vi "Initialize.vi"(8 "error in (no error)":errorcluster, 10 "timeout (ms)":u32=10000, 11 "VISA resource name":refnum<visa-resource-name>) -> (0 "error out":errorcluster, 3 "reference out":refnum<visa-resource-name>)   [LabVIEW 2012, in "USGlobalSat.lvlib"]
uses:
  USGlobalSat.lvlib
  <vilib>/Instr/_visa.llb/VISA Configure Serial Port (Instr).vi
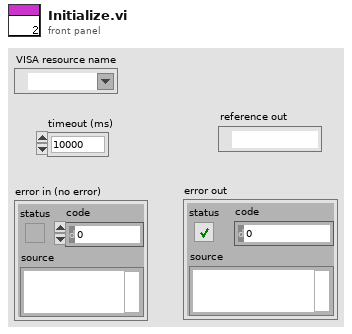
[diagram p1: front panel]
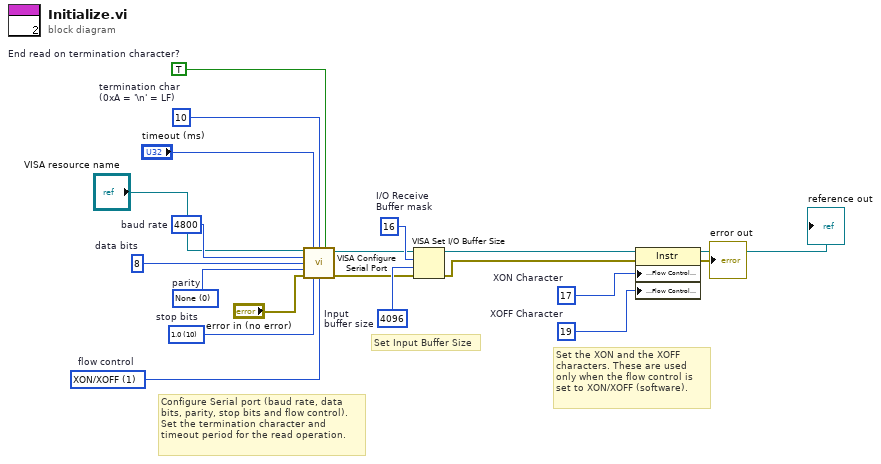
[diagram p0: block diagram]
diagram:
  w16 = TRUE  # End read on termination character?
  w8 = u8 19  # XOFF Character
  w9 = u8 17  # XON Character
  w14 = u32 4096  # Input buffer size
  w12 = u16 1 items=["None"=0, "XON/XOFF"=1, "RTS/CTS"=2, "DTR/DSR"=4]  # flow control
  w18 = u16 10 items=["1.0"=10, "1.5"=15, "2.0"=20]  # stop bits
  w19 = u16 0 items=["None", "Odd", "Even", "Mark", "Space"]  # parity
  w7 = u16 8  # data bits
  w20 = u32 4800  # baud rate
  w13 = u8 10  # termination char (0xA = '\n' = LF)
  w15 = u16 16  # I/O Receive Buffer mask
  # "Set the XON and the XOFF\ncharacters. These are used\nonly when the flow control is\nset to XON/XOFF (software)."
  # "Configure Serial port (baud rate, data\nbits, parity, stop bits and flow control).\nSet the termination character and\ntimeout period for the read operation."
  # "Set Input Buffer Size"
  n1 = call-poly "VISA Configure Serial Port"("VISA resource name"="VISA resource name", "timeout (10sec)"="timeout (ms)", "termination char\n(0xA = '\\n' = LF)"=w13, "Enable Termination\nChar (T)"=w16, "baud rate (9600)"=w20, "data bits (8)"=w7, "parity (0:none)"=w19, "error in (no error)"="error in (no error)", "stop bits (10: 1 bit)"=w18, "flow control (0:none)"=w12) -> ("VISA resource name out"=w5:refnum<visa-resource-name>, "error out"=w4:errorcluster)  [unwired: 4 in]
  n2 = VISA Set I/O Buffer Size(VISA resource name=w5, mask (16)=w15, size (4096)=w14, error in (no error)=w4) -> (VISA resource name out=w11:refnum<visa-resource-name>, error out=w10:errorcluster)
  n3 = property class="Instr"(reference=w11, error in=w10, "Serial Settings:Flow Control XON Character"=w9, "Serial Settings:Flow Control XOFF Character"=w8) -> (reference out=→"reference out":refnum<visa-resource-name>, error out=→"error out":errorcluster)
